vi "client.vi"(8 "error in (no error)":errorcluster, 11 "RemoteAnalysisToolKit in":refnum<class "RemoteAnalysisToolKit.lvclass">) -> (0 "error out":errorcluster, 3 "RemoteAnalysisToolKit out":refnum<class "RemoteAnalysisToolKit.lvclass">)   [LabVIEW 2010, in "RemoteAnalysisToolKit.lvclass"]
uses:
  RemoteAnalysisToolKit.lvclass
  RemoteAnalysisToolKit.lvclass/RemoteAnalysisToolKit.ctl
panel:
  out "Array":string[](array[string])
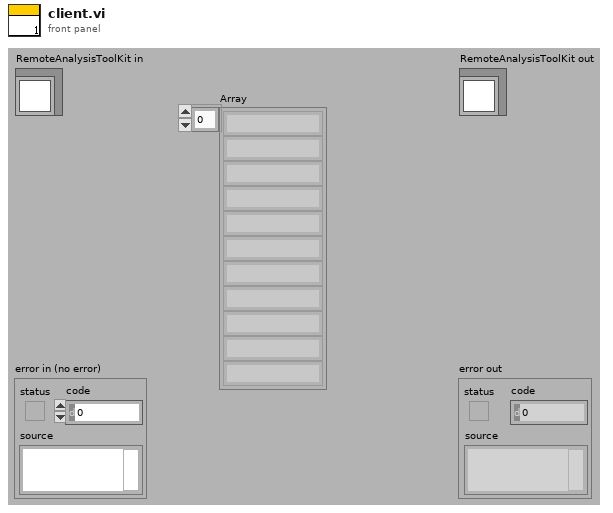
[diagram p1: front panel]
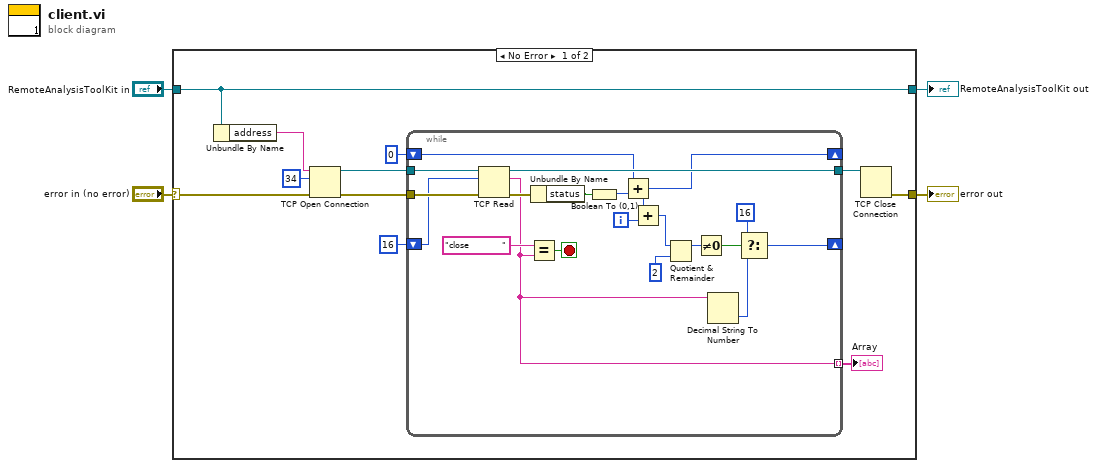
[diagram p0: block diagram]
diagram:
  n1 = case shown="No Error" "error in (no error)" {
    selector: "error in (no error)" -> [w6 w36]
    tunnel: "RemoteAnalysisToolKit in" -> [w15 w37]
    tunnel: [w7 w36] -> w2
    tunnel: [w15 w37] -> w1
    frame No Error {
      n2 = Unbundle By Name(w15) -> ("address"=w14:string)
      n3 = TCP Open Connection(address=w14, remote port or service name=u16 34, error in (no error)=w6) -> (connection ID=w12:refnum<k5>, error out=w11:errorcluster)  [unwired: 2 in]
      n4 = while {
        tunnel: w12 -> [w35]
        tunnel: w11 -> [w34]
        tunnel: [w33] -> w10
        shift-right: [w24] -> _
        shift-left: 16 -> [w30]
        shift-right: [w19] -> _
        shift-left: 0 -> [w20]
        tunnel: [w16] -> w5 mode=indexing
        i -> [w18]
        stop <- w31 stop-if-true
        n5 = TCP Read(connection ID=w35, bytes to read=w30, error in (no error)=w34) -> (connection ID out=w33:refnum<k5>, data out=w16:string, error out=w23:errorcluster)  [unwired: 2 in]
        n6 = Equal?(x="close           " ("data in"), y=w16) -> (x = y?=w31:bool)
        n7 = Unbundle By Name(w23) -> ("status"=w22:bool)
        n8 = Boolean To (0,1)(Boolean=w22) -> (0, 1=w21:i16)
        n9 = Add(x=w20, y=w21) -> (x+y=w19:i32)
        n10 = Add(x=w19, y=w18) -> (x+y=w17:i32)
        n11 = Quotient & Remainder(x=w17, y=2) -> (x-y*floor(x/y)=w27:i32)  [unwired: 1 out]
        n12 = Not Equal To 0?(x=w27) -> (x != 0?=w28:bool)
        n13 = Decimal String To Number(string=w16) -> (number=w25:i32)  [unwired: 2 in, 1 out]
        n14 = Select(t=16, s=w28, f=w25) -> (s? t:f=w24:i32)
      }
      "Array" <- w5
      n15 = TCP Close Connection(connection ID=w10) -> (error out=w7:errorcluster)  [unwired: 2 in, 1 out]
    }
    frame Error {
    }
  }
  "error out" <- w2
  "RemoteAnalysisToolKit out" <- w1
